vi "Create Pattern Script(DataCompare).vi"(8 "error in (no error)":errorcluster, 9 "Data":u8[](array[numeric]), 10 "Num of wait cycle for read":i8, 11 "BML Pattern Creater in":refnum<class "BML Pattern Creater.lvclass">) -> (0 "error out":errorcluster, 2 "String":string, 3 "BML Pattern Creater out":refnum<class "BML Pattern Creater.lvclass">)   [LabVIEW 2018, in "BML Pattern Creater.lvlib" / "BML Pattern Creater.lvclass"]
uses:
  BML Pattern Creater.lvclass
  Interfaces/Protocol Interface.lvlibp/Interfaces/Protocol Interface/Pin State.ctl
  Interfaces/Protocol Interface.lvlibp/Interfaces/Protocol Interface/Protocol Interface.lvclass
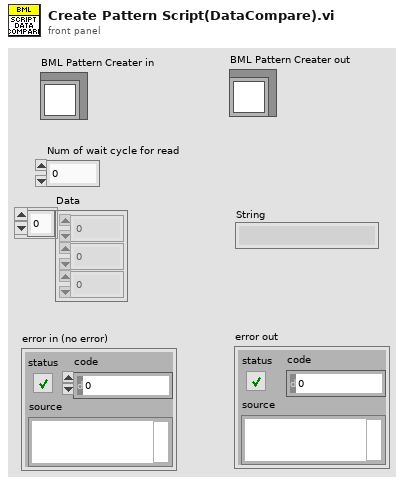
[diagram p1: front panel]
types:
  T1 = typedef "Protocol Interface.lvlibp/Protocol Interface.lvclass/Pin State.ctl" = enum16{"0", "1", "L", "H", "X", "V", "D", "M"}
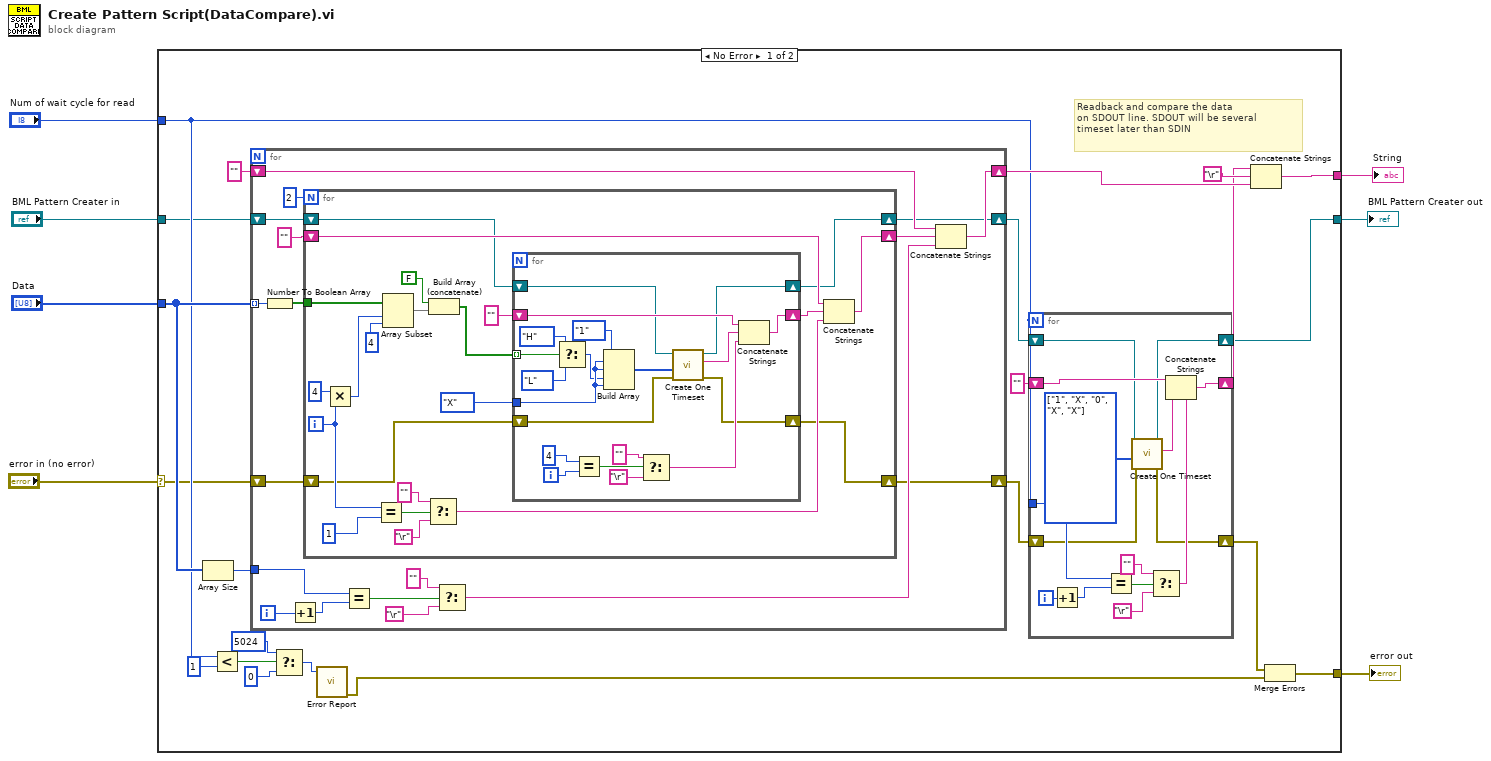
[diagram p0: block diagram]
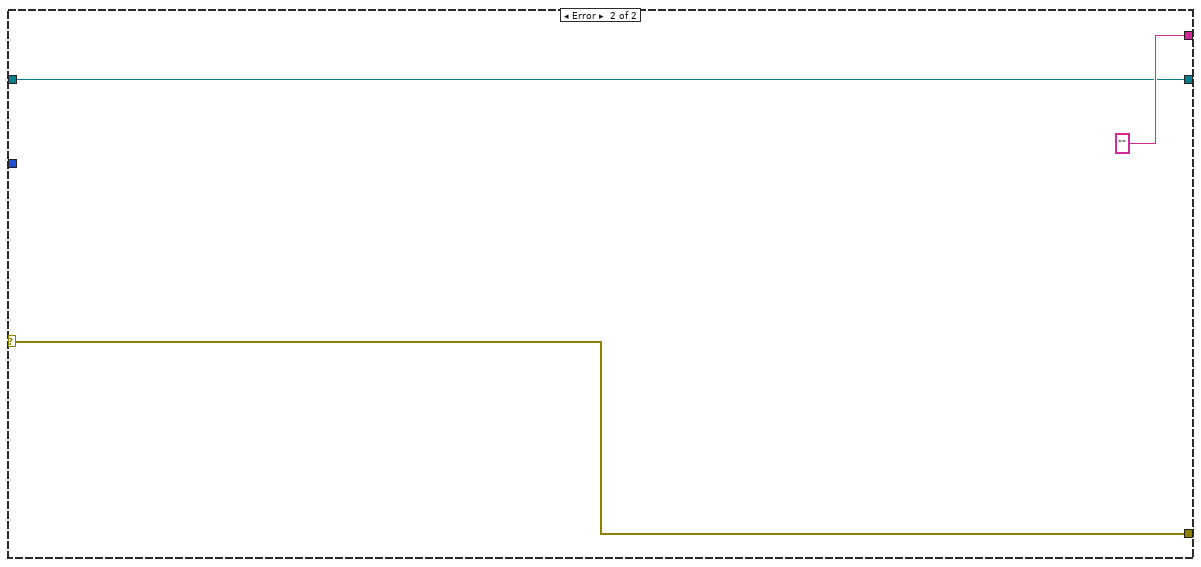
[diagram p2: hidden frame]
diagram:
  n1 = case shown="No Error" "error in (no error)" {
    selector: "error in (no error)" -> [w15 w106]
    tunnel: [w24 ""] -> w6
    tunnel: [w9 w106] -> w5
    tunnel: "Data" -> [w29 _]
    tunnel: "Num of wait cycle for read" -> [w16 _]
    tunnel: "BML Pattern Creater in" -> [w14 w105]
    tunnel: [w8 w105] -> w1
    frame No Error {
      # "Readback and compare the data\non SDOUT line. SDOUT will be several \ntimeset later than SDIN"
      n2 = Array Size(array=w29) -> (size(s)=w28:i32)
      n3 = Less?(x=w16, y=i8 1) -> (x < y?=w18:bool)
      n4 = for {
        tunnel: w29 -> [w59] mode=indexing
        tunnel: w28 -> [w56]
        shift-right: [w50] -> w25
        shift-left: "" -> [w49]
        shift-right: [w47] -> w13
        shift-left: w15 -> [w48]
        shift-right: [w45] -> w12
        shift-left: w14 -> [w46]
        i -> [w58]
        n5 = Number To Boolean Array(number=w59) -> (Boolean array=w62:bool[])
        n6 = Increment(x=w58) -> (x+1=w57:i32)
        n7 = for {
          N: 2 -> [_]
          tunnel: w62 -> [w84]
          shift-right: [w69] -> w52
          shift-left: "" -> [w68]
          shift-right: [w65] -> w47
          shift-left: w48 -> [w66]
          shift-right: [w63] -> w45
          shift-left: w46 -> [w64]
          i -> [w76]
          n8 = Multiply(x=4 ("y"), y=w76) -> (x*y=w82:i32)
          n9 = Equal?(x=w76, y=1) -> (x = y?=w74:bool)
          n10 = Array Subset(array=w84, index=w82, length=4) -> (w81:bool[])
          n11 = Select(t="", s=w74, f="\r") -> (s? t:f=w70:string)
          n12 = Build Array (concatenate)(FALSE, w81) -> (w78:bool[])
          n13 = for {
            tunnel: w78 -> [w104] mode=indexing
            shift-right: [w98] -> w71
            shift-left: "" -> [w97]
            tunnel: Pin_State."X" ("PinState") -> [w95]
            shift-right: [w87] -> w65
            shift-left: w66 -> [w88]
            shift-right: [w85] -> w63
            shift-left: w64 -> [w86]
            i -> [w103]
            n14 = Select(t=Pin_State."H" ("PinState"), s=w104, f=Pin_State."L" ("PinState")) -> (s? t:f=w94:T1)
            n15 = Equal?(x=4, y=w103) -> (x = y?=w101:bool)
            n16 = Build Array(Pin_State."1" ("PinState"), w95, w95, w94, w95) -> (w93:T1[])
            n17 = Select(t="", s=w101, f="\r") -> (s? t:f=w96:string)
            n18 = call-dynamic "Create One Timeset.vi"("error in (no error)"=w88, "Pin State"=w93, "BML Pattern Creater in"=w86) -> ("error out"=w87:errorcluster, "string out"=w92:string, "BML Pattern Creater out"=w85:refnum<class "BML Pattern Creater.lvclass">)  [unwired: 6 in]
            n19 = Concatenate Strings(w97, w92, w96) -> (w98:string)
          }
          n20 = Concatenate Strings(w68, w71, w70) -> (w69:string)
        }
        n21 = Equal?(x=w56, y=w57) -> (x = y?=w53:bool)
        n22 = Select(t="", s=w53, f="\r") -> (s? t:f=w51:string)
        n23 = Concatenate Strings(w49, w52, w51) -> (w50:string)
      }
      n24 = Select(t=i16 5024, s=w18, f=i16 0 ("Error Code")) -> (s? t:f=w21:i16)
      n25 = call "Error Report.vi"("Error Code"=w21) -> ("error out"=w10:errorcluster)  [unwired: 10 in]
      n26 = for {
        N: w16 -> [_]
        shift-right: [w44] -> w22
        shift-left: "" -> [w43]
        tunnel: w16 -> [w37]
        shift-right: [w32] -> w11
        shift-left: w13 -> [w33]
        shift-right: [w30] -> w8
        shift-left: w12 -> [w31]
        i -> [w38]
        w34 = T1[] [enum."1", enum."X", enum."0", enum."X", enum."X"] items=["0", "1", "L", "H", "X", "V", "D", "M"] ("Array")
        n27 = Increment(x=w38) -> (x+1=w42:i32)
        n28 = Equal?(x=w37, y=w42) -> (x = y?=w39:bool)
        n29 = call-dynamic "Create One Timeset.vi"("error in (no error)"=w33, "Pin State"=w34, "BML Pattern Creater in"=w31) -> ("error out"=w32:errorcluster, "string out"=w35:string, "BML Pattern Creater out"=w30:refnum<class "BML Pattern Creater.lvclass">)  [unwired: 6 in]
        n30 = Select(t="", s=w39, f="\r") -> (s? t:f=w36:string)
        n31 = Concatenate Strings(w43, w35, w36) -> (w44:string)
      }
      n32 = Concatenate Strings(w22, "\r", w25) -> (w24:string)
      n33 = Merge Errors(w11, w10) -> (w9:errorcluster)
    }
    frame Error {
    }
  }
  "String" <- w6
  "error out" <- w5
  "BML Pattern Creater out" <- w1
